vi "Calculate time scaling parameters.vi"(5 "Time":i64, 7 "Time scale (minutes)":i64) -> (0 "Minimum":dbl, 1 "Maximum":dbl, 2 "Increment":dbl, 3 "Minor increment":dbl, 4 "Start":dbl)   [LabVIEW 2019]
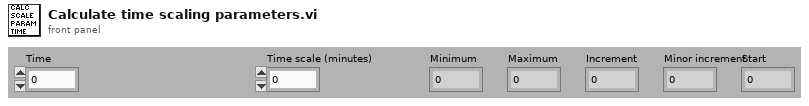
[diagram p1: front panel]
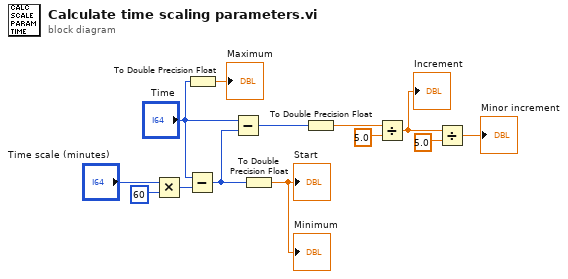
[diagram p0: block diagram]
diagram:
  n1 = Multiply(x="Time scale (minutes)", y=i64 60) -> (x*y=w13:i64)
  n2 = Subtract(x="Time", y=w13) -> (x-y=w9:i64)
  n3 = To Double Precision Float(number="Time") -> (double precision float=→"Maximum":dbl)
  n4 = Subtract(x="Time", y=w9) -> (x-y=w7:i64)
  n5 = To Double Precision Float(number=w9) -> (double precision float=→"Start" →"Minimum":dbl)
  n6 = To Double Precision Float(number=w7) -> (double precision float=w8:dbl)
  n7 = Divide(x=w8, y=5.0) -> (x/y=w10:dbl)
  "Increment" <- w10
  n8 = Divide(x=w10, y=5.0) -> (x/y=→"Minor increment":dbl)
